vi "Read Parameters to process.vi"(8 "error in":errorcluster, 11 "Custom Temperature Controller runtime in":refnum<class "Custom Temperature Controller runtime.lvclass">) -> (0 "error out":errorcluster, 2 "Parameters to process":T1, 3 "Custom Temperature Controller runtime out":refnum<class "Custom Temperature Controller runtime.lvclass">)   [LabVIEW 2021, in "Custom Temperature Controller runtime.lvclass"]
uses:
  Custom Temperature Controller runtime.lvclass
  configuration/parameter data indices.ctl
  Custom Temperature Controller runtime.lvclass/Custom Temperature Controller runtime.ctl
  configuration/Custom Temperature Controller configuration.lvclass
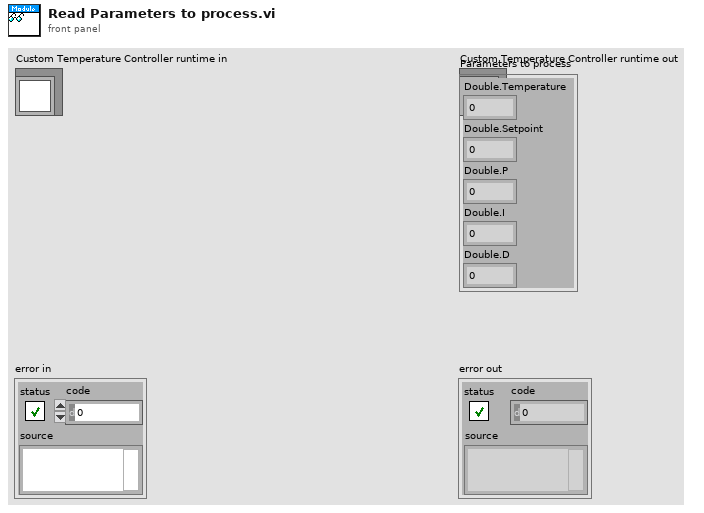
[diagram p1: front panel]
types:
  T1 = typedef "Custom Temperature Controller configuration.lvclass/parameter data indices.ctl" = cluster{"Double.Temperature":i32, "Double.Setpoint":i32, "Double.P":i32, "Double.I":i32, "Double.D":i32}
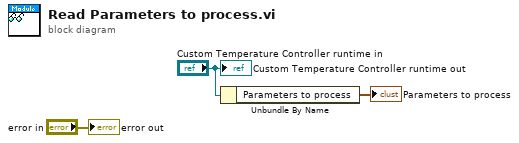
[diagram p0: block diagram]
diagram:
  n1 = Unbundle By Name("Custom Temperature Controller runtime in") -> ("Parameters to process"=→"Parameters to process":T1)
  "error out" <- "error in"
  "Custom Temperature Controller runtime out" <- "Custom Temperature Controller runtime in"
